vi "pwm.vi"() -> ()   [LabVIEW 2010]
uses:
  libdaqVI.lvlib
panel:
  in  "退出程序":bool
  in  "选项卡控件":enum32{"PWM1", "PWM2"}(tab)
  in  "pwm1_set":bool
  in  "pwm1_start":bool
  in  "pwm1_stop":bool
  in  "period":u32=1000000 caption="周期(ns)"
  in  "pulse":u32=500000 caption="脉冲宽度(ns)"
  in  "脉冲数":u32
  in  "pwm2_stop":bool
  in  "pwm2_start":bool
  in  "pwm2_set":bool
  in  "period 2":u32=1000000 caption="周期(ns)"
  in  "pulse 2":u32=500000 caption="脉冲宽度(ns)"
  in  "脉冲数":i32
  out "状态":bool
  out "设备名称":string
  out "设备数量":u32
  # "范例说明：\n1、支持的采集卡：DAQ-USB3212、DAQ-USB3213、DAQ-USB3214\n2、PWM1和PWM2模块，包括PWM发生和脉冲发生两种模式，当脉冲数为0时，为连续PWM发生模式，脉冲数不为0时，为脉冲发生模式，脉冲数的值即为脉冲的个数；\n\n注意：\n1、脉冲发生模式会产生单片机中断，因此脉冲频率不建议超过10kHz；PWM发送器无需单片机干预，可以支持到1MHz；\n2、ADC模块的波形采样、DAC模块的波形输出工作过程也会产生单片机的中断，当单片机中断过于频繁会造成上位机下发的指令得不到响应，采集卡死机的假象，因此当与这些模块同时使用时，COUNTER模块、PWM模块、ADC和DAC模块的工作频率需要进一步降低；\n3、采集卡包含ADC、DAC、CNT1、CNT2、PWM1、PWM2总共6个模块，建议同时使用的模块不要超过3个，具体以测试为准\n4、PWM模块中周期和脉冲宽度的单位为纳秒(ns)"
  # "计数模块演示程序"
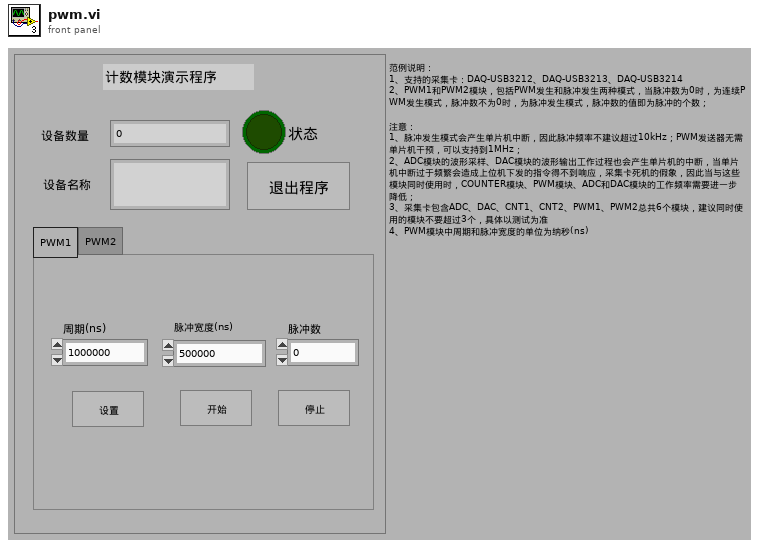
[diagram p1: front panel]
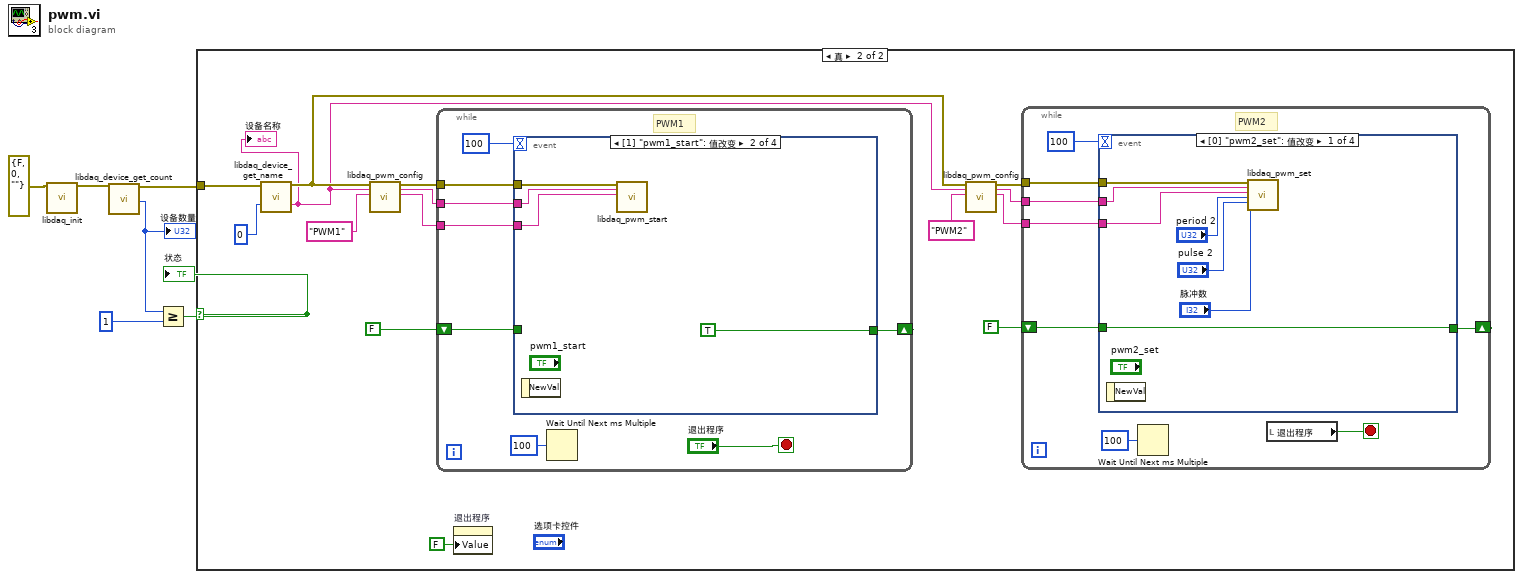
[diagram p0: block diagram]
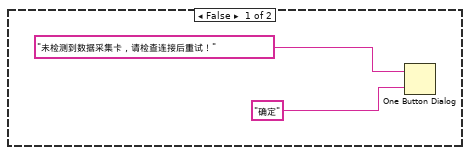
[diagram p2: hidden frame]
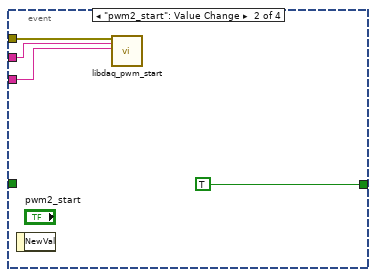
[diagram p3: hidden frame]
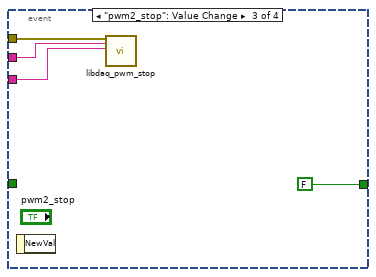
[diagram p4: hidden frame]
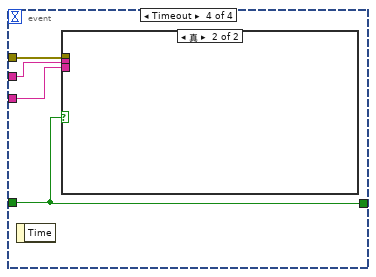
[diagram p5: hidden frame]
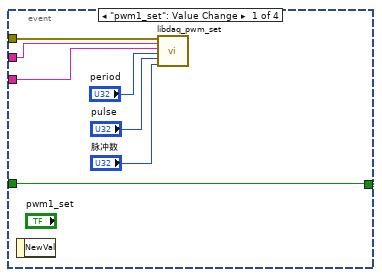
[diagram p7: hidden frame]
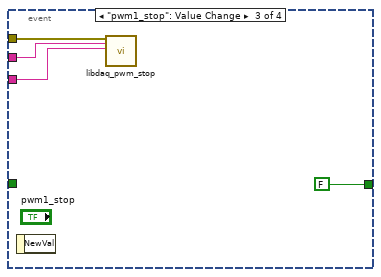
[diagram p8: hidden frame]
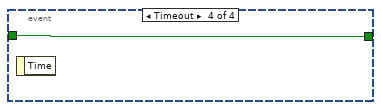
[diagram p9: hidden frame]
diagram:
  n1 = call "libdaq_init.vi"("error in (no error)"=errorcluster {"status"=FALSE, "code"=0, "source"=""}) -> ("error out"=w2:errorcluster)  [unwired: 18 in]
  n2 = call "libdaq_device_get_count.vi"("error in (no error)"=w2) -> ("error out"=w3:errorcluster, "device_count"=w1:i32)  [unwired: 17 in]
  "设备数量" <- w1
  n3 = Greater Or Equal?(x=w1, y=u32 1 ("name length")) -> (x >= y?=w5:bool)
  "状态" <- w5
  n4 = case shown="真" w5 {
    tunnel: w3 -> [_ w23]
    frame False {
      n5 = One Button Dialog(message="未检测到数据采集卡，请检查连接后重试！" ("消息"), button name ("OK")="确定" ("按钮名称（“确定”）")) -> ()  [unwired: 1 out]
    }
    frame True {
      n6 = call "libdaq_device_get_name.vi"("error in (no error)"=w23, "device_index"=u32 0 ("name length")) -> ("error out"=w14:errorcluster, "device_name"=w12:string)  [unwired: 16 in]
      "设备名称" <- w12
      n7 = call "libdaq_pwm_config.vi"("error in (no error)"=w14, "device_name"=w12, "module_name"="PWM1") -> ("error out"=w18:errorcluster, "device_name"=w17:string, "module_name"=w16:string)  [unwired: 14 in]
      n8 = while {
        tunnel: w18 -> [w57]
        tunnel: w17 -> [w56]
        shift-right: [w54] -> _
        shift-left: FALSE -> [w55]
        tunnel: w16 -> [w51]
        stop <- "退出程序" stop-if-true
        # "PWM1"
        n9 = event shown="[1] \"pwm1_start\": 值改变" {
          selector: _ -> [_ _ _ _]
          dyn-events: _ -> [_ _ _ _]
          timeout: 100 -> [_ _ _ _]
          tunnel: w57 -> [w65 w69 w73 _]
          tunnel: w56 -> [w64 w68 w72 _]
          tunnel: w51 -> [w63 w67 w71 _]
          tunnel: w55 -> [w62 _ _ w74]
          tunnel: [w62 TRUE FALSE w74] -> w54
          event "pwm1_set": Value Change {
            n10 = event-data() -> ()  [unwired: 1 in, 1 out]
            n11 = call "libdaq_pwm_set.vi"("error in (no error)"=w65, "device_name"=w64, "module_name"=w63, "period"="period", "pulse"="pulse", "count"="脉冲数") -> ()  [unwired: 11 in, 3 out]
          }
          event "pwm1_start": Value Change {
            n12 = event-data() -> ()  [unwired: 1 in, 1 out]
            n13 = call "libdaq_pwm_start.vi"("error in (no error)"=w69, "device_name"=w68, "module_name"=w67) -> ()  [unwired: 14 in, 3 out]
          }
          event "pwm1_stop": Value Change {
            n14 = event-data() -> ()  [unwired: 1 in, 1 out]
            n15 = call "libdaq_pwm_stop.vi"("error in (no error)"=w73, "device_name"=w72, "module_name"=w71) -> ()  [unwired: 14 in, 3 out]
          }
          event Timeout {
            n16 = event-data() -> ()  [unwired: 1 in, 1 out]
          }
        }
        n17 = Wait Until Next ms Multiple(millisecond multiple=u32 100 ("毫秒倍数")) -> ()  [unwired: 1 out]
      }
      n18 = property on="退出程序" class="Bool (严格)"("Value"=FALSE ("退出程序")) -> ()  [unwired: 2 in, 2 out]
      n19 = call "libdaq_pwm_config.vi"("error in (no error)"=w14, "device_name"=w12, "module_name"="PWM2") -> ("error out"=w13:errorcluster, "device_name"=w11:string, "module_name"=w10:string)  [unwired: 14 in]
      n20 = while {
        tunnel: w13 -> [w30]
        tunnel: w11 -> [w29]
        shift-right: [w27] -> _
        shift-left: FALSE -> [w28]
        tunnel: w10 -> [w24]
        stop <- w26 stop-if-true
        # "PWM2"
        n21 = event shown="[0] \"pwm2_set\": 值改变" {
          selector: _ -> [_ _ _ _]
          dyn-events: _ -> [_ _ _ _]
          timeout: 100 -> [_ _ _ _]
          tunnel: w30 -> [w38 w42 w46 w50]
          tunnel: w29 -> [w37 w41 w45 w49]
          tunnel: w24 -> [w36 w40 w44 w48]
          tunnel: w28 -> [w35 _ _ w47]
          tunnel: [w35 TRUE FALSE w47] -> w27
          event "pwm2_set": Value Change {
            n22 = event-data() -> ()  [unwired: 1 in, 1 out]
            n23 = call "libdaq_pwm_set.vi"("error in (no error)"=w38, "device_name"=w37, "module_name"=w36, "period"="period 2", "pulse"="pulse 2", "count"="脉冲数") -> ()  [unwired: 11 in, 3 out]
          }
          event "pwm2_start": Value Change {
            n24 = event-data() -> ()  [unwired: 1 in, 1 out]
            n25 = call "libdaq_pwm_start.vi"("error in (no error)"=w42, "device_name"=w41, "module_name"=w40) -> ()  [unwired: 14 in, 3 out]
          }
          event "pwm2_stop": Value Change {
            n26 = event-data() -> ()  [unwired: 1 in, 1 out]
            n27 = call "libdaq_pwm_stop.vi"("error in (no error)"=w46, "device_name"=w45, "module_name"=w44) -> ()  [unwired: 14 in, 3 out]
          }
          event Timeout {
            n28 = event-data() -> ()  [unwired: 1 in, 1 out]
            n29 = case shown="真" w47 {
              tunnel: w50 -> [_ _]
              tunnel: w49 -> [_ _]
              tunnel: w48 -> [_ _]
              frame False {
              }
              frame True {
              }
            }
          }
        }
        n30 = Wait Until Next ms Multiple(millisecond multiple=u32 100 ("毫秒倍数")) -> ()  [unwired: 1 out]
        n31 = local read "退出程序"() -> (w26:bool)
      }
    }
  }
